vi "solar_qtimer Daemon.vi"(10 "Instance":i32, 11 "QTimerRefnum":T1) -> (0 "error out":errorcluster)   [LabVIEW 2018]
doc: "This is the spawned daemon to periodically enqueue commands."
uses:
  solar_qtimer_ctl Refnum.ctl
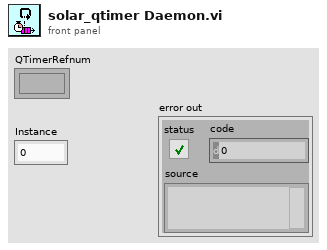
[diagram p1: front panel]
types:
  T1 = typedef "solar_qtimer_ctl Refnum.ctl" = refnum<k1>
  T2 = typedef "solar_qtimer_ctl QTimer.ctl" = cluster{"Settings":T3, "Queue":refnum<queue>, "QTimerQ":refnum<queue>, "VI Refnum":refnum<vi>}
  T3 = typedef "solar_qtimer_ctl QTimer Settings.ctl" = cluster{"QTimer":string, "Delay":i32, "Start":bool, "EnQ_Type":enum8{"Normal", "Priority", "IgnoreIfExists"}, "Messages":cluster{"MSG":string, "DATA":variant}[]}
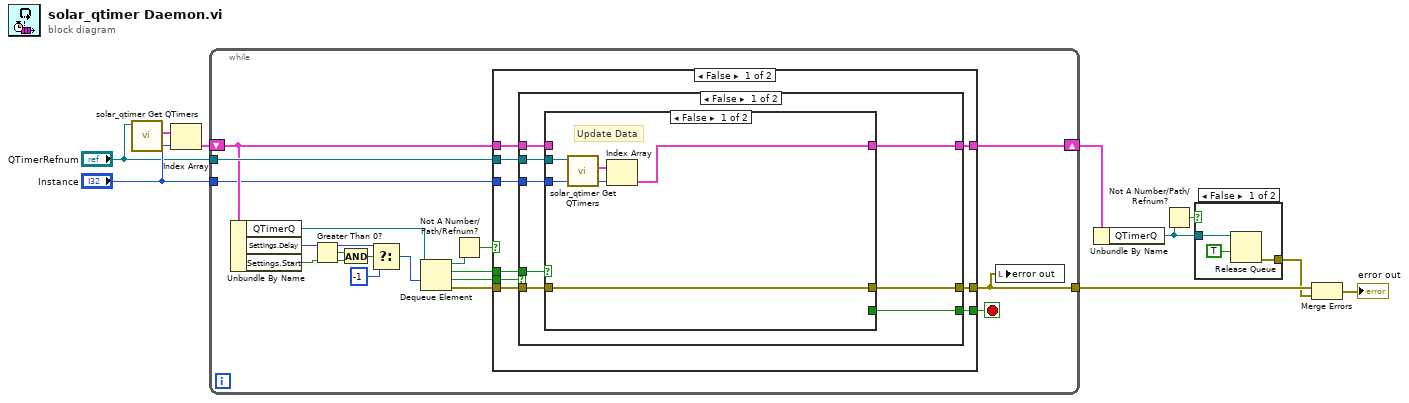
[diagram p0: block diagram]
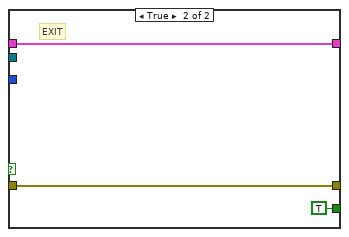
[diagram p3: hidden frame]
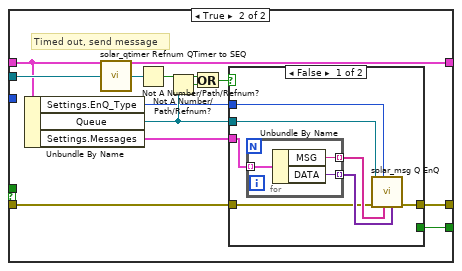
[diagram p4: hidden frame]
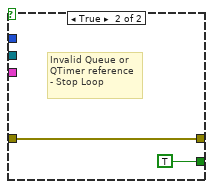
[diagram p5: hidden frame]
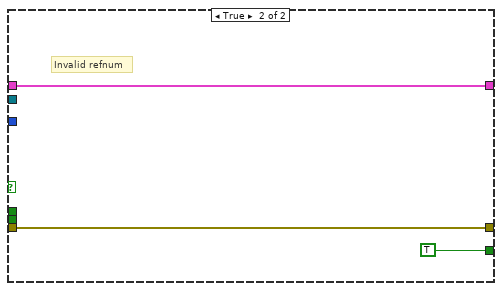
[diagram p6: hidden frame]
diagram:
  n1 = call "solar_qtimer Get QTimers.vi"("QTimer Refnum"="QTimerRefnum") -> ("QTimers"=w8:T2[])  [unwired: 8 in, 2 out]
  n2 = Index Array(array=w8, index="Instance") -> (element=w7:T2)
  n3 = while {
    shift-right: [w14] -> w5
    shift-left: w7 -> [w19]
    tunnel: "QTimerRefnum" -> [w20]
    tunnel: "Instance" -> [w15]
    tunnel: [w11] -> w6
    stop <- w13 stop-if-true
    n4 = Unbundle By Name(w19) -> ("QTimerQ"=w22:refnum<queue>, "Settings.Delay"=w25:i32, "Settings.Start"=w27:bool)
    n5 = Greater Than 0?(x=w25) -> (x > 0?=w28:bool)
    n6 = And(x=w28, y=w27) -> (x .and. y?=w26:bool)
    n7 = Select(t=w25, s=w26, f=-1) -> (s? t:f=w23:i32)
    n8 = Dequeue Element(queue=w22, timeout in ms (-1)=w23) -> (queue out=w16:refnum<queue>, element=w17:bool, timed out?=w18:bool, error out=w21:errorcluster)  [unwired: 1 in]
    n9 = Not A Number/Path/Refnum?(number/path/refnum=w16) -> (NaN/Path/Refnum?=w12:bool)
    n10 = case shown="False" w12 {
      tunnel: w21 -> [w37 w79]
      tunnel: w20 -> [w36 _]
      tunnel: w19 -> [w35 w80]
      tunnel: w18 -> [w34 _]
      tunnel: w17 -> [w33 _]
      tunnel: w15 -> [w32 _]
      tunnel: [w31 w80] -> w14
      tunnel: [w30 w79] -> w11
      tunnel: [w29 TRUE] -> w13
      frame False {
        n11 = case shown="False" w34 {
          tunnel: w37 -> [w43 w59]
          tunnel: w36 -> [w41 w58]
          tunnel: w35 -> [w39 w56]
          tunnel: [w44 w54] -> w29
          tunnel: w33 -> [w45 _]
          tunnel: [w42 w57] -> w30
          tunnel: w32 -> [w40 _]
          tunnel: [w38 w56] -> w31
          frame False {
            n12 = case shown="False" w45 {
              tunnel: [_ TRUE] -> w44
              tunnel: w43 -> [w46 w51]
              tunnel: [w46 w51] -> w42
              tunnel: w41 -> [w49 _]
              tunnel: w40 -> [w48 _]
              tunnel: w39 -> [_ w52]
              tunnel: [w47 w52] -> w38
              frame False {
                # "Update Data"
                n13 = call "solar_qtimer Get QTimers.vi"("QTimer Refnum"=w49) -> ("QTimers"=w50:T2[])  [unwired: 8 in, 2 out]
                n14 = Index Array(array=w50, index=w48) -> (element=w47:T2)
              }
              frame True {
                # "EXIT"
              }
            }
          }
          frame True {
            # "Timed out, send message"
            n15 = Unbundle By Name(w56) -> ("Settings.EnQ_Type"=w61:enum8{"Normal", "Priority", "IgnoreIfExists"}, "Queue"=w63:refnum<queue>, "Settings.Messages"=w60:cluster{"MSG":string, "DATA":variant}[])
            n16 = call "solar_qtimer Refnum QTimer to SEQ.vi"("QTimer Refnum"=w58) -> ("QTimers SEQ"=w62:refnum<queue>)
            n17 = Not A Number/Path/Refnum?(number/path/refnum=w62) -> (NaN/Path/Refnum?=w64:bool)
            n18 = Not A Number/Path/Refnum?(number/path/refnum=w63) -> (NaN/Path/Refnum?=w65:bool)
            n19 = Or(x=w64, y=w65) -> (x .or. y?=w55:bool)
            n20 = case shown="False" w55 {
              tunnel: w63 -> [w72 _]
              tunnel: w61 -> [w71 _]
              tunnel: w60 -> [w68 _]
              tunnel: w59 -> [w67 w77]
              tunnel: [w66 w77] -> w57
              tunnel: [_ TRUE] -> w54
              frame False {
                n21 = for {
                  tunnel: w68 -> [w75] mode=indexing
                  tunnel: [w74] -> w69 mode=indexing
                  tunnel: [w73] -> w70 mode=indexing
                  n22 = Unbundle By Name(w75) -> ("MSG"=w74:string, "DATA"=w73:variant)
                }
                n23 = call "solar_msg Q EnQ.vi"("CMD_DATA Array"=w70, "CMD Array"=w69, "Priority (Normal)"=w71, "error in (no error)"=w67, "Queue in"=w72) -> ("error out"=w66:errorcluster)  [unwired: 4 in, 2 out]
              }
              frame True {
                # "Invalid Queue or\nQTimer reference\n- Stop Loop"
              }
            }
          }
        }
      }
      frame True {
        # "Invalid refnum"
      }
    }
    n24 = local write "error out"(w11) -> ()
  }
  n25 = Unbundle By Name(w5) -> ("QTimerQ"=w2:refnum<queue>)
  n26 = Not A Number/Path/Refnum?(number/path/refnum=w2) -> (NaN/Path/Refnum?=w1:bool)
  n27 = case shown="False" w1 {
    tunnel: w2 -> [w82 _]
    tunnel: [w81 _] -> w3
    frame False {
      n28 = Release Queue(queue=w82, force destroy? (F)=TRUE) -> (error out=w81:errorcluster)  [unwired: 1 in, 2 out]
    }
    frame True {
    }
  }
  n29 = Merge Errors(w6, w3) -> (→"error out":errorcluster)
